vi "NewLifetimeForRobot.vi"(10 "Last robots":T1[](array[typedef]) {"height" format="%+4.3f"; "pixel_y" format="%+4.3f"; "pixel_x" format="%+4.3f"; "orientation" format="%+4.3f"; "y" format="%+4.3f"; "confidence" format="%4.3f"; "x" format="%+4.3f"}, 11 "Current robots":T1[](array[typedef]) {"height" format="%+4.3f"; "pixel_y" format="%+4.3f"; "pixel_x" format="%+4.3f"; "orientation" format="%+4.3f"; "y" format="%+4.3f"; "confidence" format="%4.3f"; "x" format="%+4.3f"}) -> (3 "Array of robots":T1[](array[typedef]) {"height" format="%+4.3f"; "pixel_y" format="%+4.3f"; "pixel_x" format="%+4.3f"; "orientation" format="%+4.3f"; "y" format="%+4.3f"; "confidence" format="%4.3f"; "x" format="%+4.3f"})   [LabVIEW 2023]
uses:
  Old vision/Controls/SSL Detection Robot.ctl
  <vilib>/Analysis/Matrix/Datatypes/RealMatrix.ctl
  <vilib>/Analysis/Matrix/NI_Matrix.lvlib
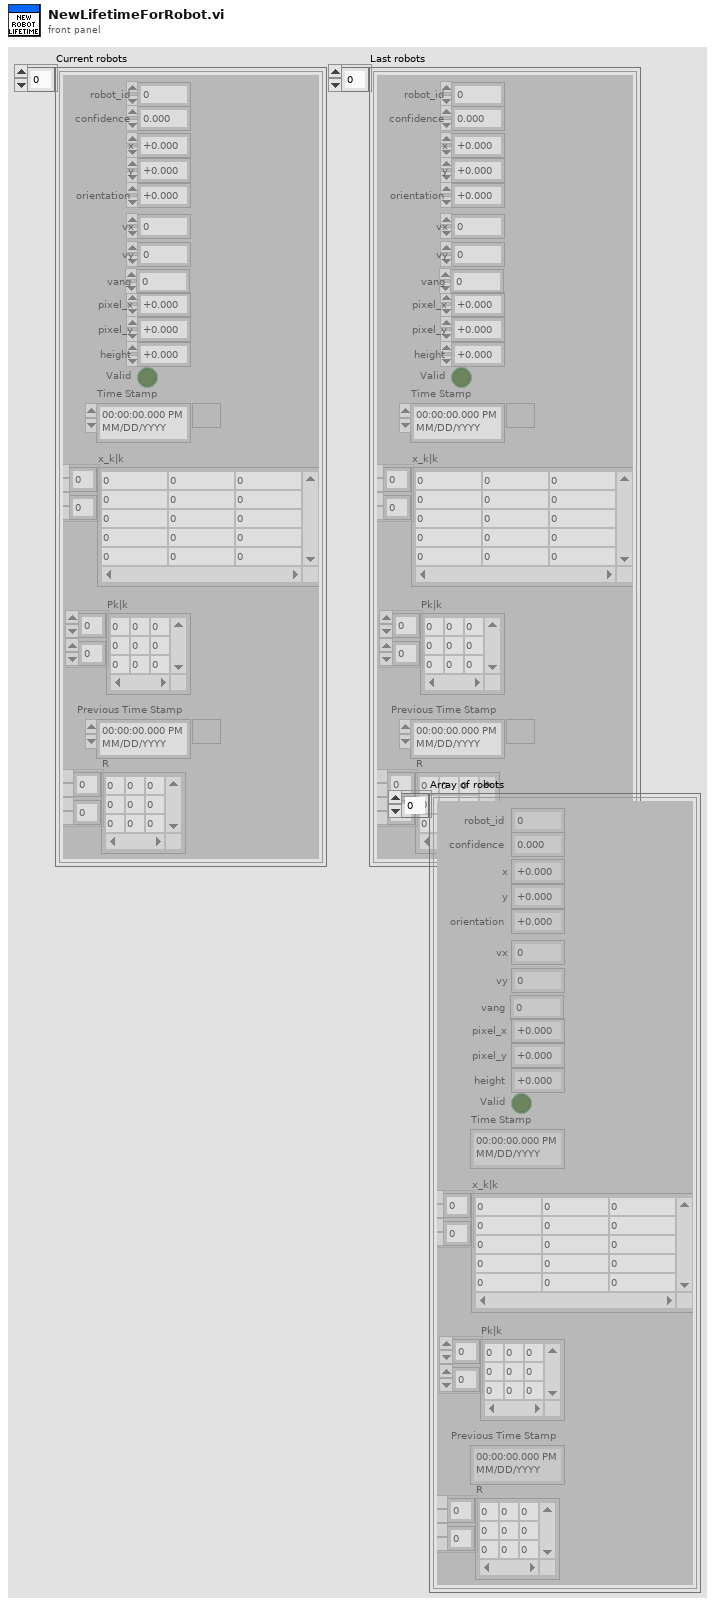
[diagram p1: front panel]
types:
  T1 = typedef "SSL Detection Robot.ctl" = cluster{"x":sgl, "robot_id":u32, "confidence":sgl, "y":sgl, "orientation":sgl, "pixel_x":sgl, "pixel_y":sgl, "height":sgl, "Valid":bool, "Time Stamp":timestamp, "x_k|k":T2, "Pk|k":T2, "Previous Time Stamp":timestamp, "R":T2, "vx":dbl, "vy":dbl, "vang":dbl}
  T2 = typedef "NI_Matrix.lvlib/RealMatrix.ctl" = dbl[][]
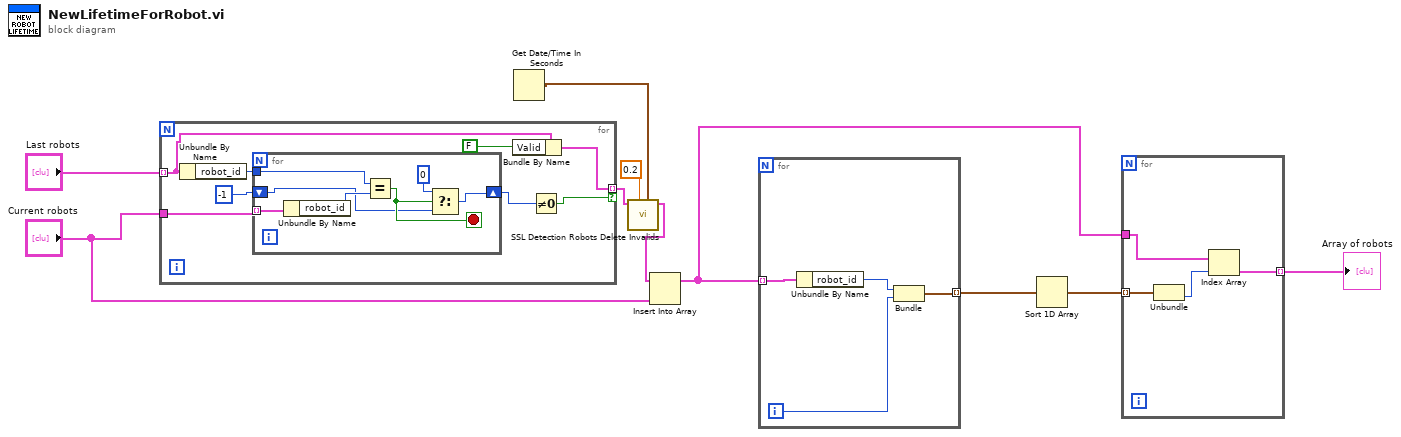
[diagram p0: block diagram]
diagram:
  n1 = for {
    tunnel: "Last robots" -> [w13] mode=indexing
    tunnel: "Current robots" -> [w18]
    tunnel: [w12] -> w4 mode=indexing if=w14
    n2 = Unbundle By Name(w13) -> ("robot_id"=w17:u32)
    n3 = for {
      tunnel: w18 -> [w25] mode=indexing
      tunnel: w17 -> [w24]
      shift-right: [w22] -> w15
      shift-left: -1 -> [w19]
      stop <- w20 stop-if-true
      n4 = Unbundle By Name(w25) -> ("robot_id"=w23:u32)
      n5 = Equal?(x=w24, y=w23) -> (x = y?=w20:bool)
      n6 = Select(t=0, s=w20, f=w19) -> (s? t:f=w22:i32)
    }
    n7 = Bundle By Name(cluster=w13, "Valid"=FALSE) -> (w12:T1)
    n8 = Not Equal To 0?(x=w15) -> (x != 0?=w14:bool)
  }
  n9 = Get Date/Time In Seconds() -> (seconds since 1Jan1904=w1:timestamp)
  n10 = call "SSL Detection Robots Delete Invalids.vi"("Now"=w1, "Life Time"=0.2, "Robots In"=w4) -> ("Robots Out"=w3:T1[])  [unwired: 8 in]
  n11 = Insert Into Array(array=w3, new element="Current robots") -> (w6:T1[])  [unwired: 1 in]
  n12 = for {
    tunnel: [w27] -> w9 mode=indexing
    tunnel: w6 -> [w26] mode=indexing
    i -> [w28]
    n13 = Unbundle By Name(w26) -> ("robot_id"=w29:u32)
    n14 = Bundle("robot_id"=w29, w28) -> (w27:cluster{"robot_id":u32, i32})  [unwired: 1 in]
  }
  n15 = Sort 1D Array(array=w9) -> (sorted array=w8:cluster{"robot_id":u32, i32}[])
  n16 = for {
    tunnel: w8 -> [w32] mode=indexing
    tunnel: w6 -> [w33]
    tunnel: [w30] -> w5 mode=indexing
    n17 = Unbundle(w32) -> (w31:i32)  [unwired: 1 out]
    n18 = Index Array(array=w33, index=w31) -> (element=w30:T1)
  }
  "Array of robots" <- w5
